vi "Cost.vi"(8 "error in (no error)":errorcluster, 11 "Dark Roast in":refnum<class "Dark Roast.lvclass">) -> (0 "error out":errorcluster, 2 "Cost":dbl, 3 "Dark Roast out":refnum<class "Dark Roast.lvclass">)   [LabVIEW 2020, in "Dark Roast.lvclass"]
uses:
  Dark Roast.lvclass
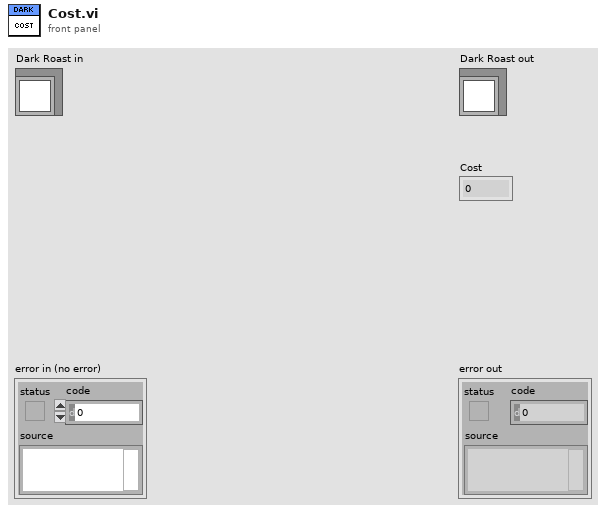
[diagram p1: front panel]
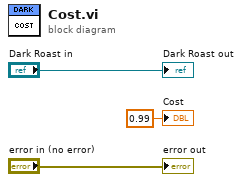
[diagram p0: block diagram]
diagram:
  "error out" <- "error in (no error)"
  "Dark Roast out" <- "Dark Roast in"
  "Cost" <- 0.99 ("Cost")
